vi "Fitts_test.vi"(11 "ID":dbl) -> (1 "W":dbl, 2 "D":dbl=1.0)   [LabVIEW 2010]
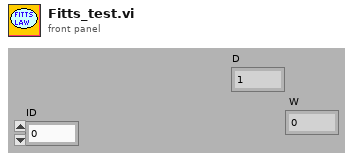
[diagram p1: front panel]
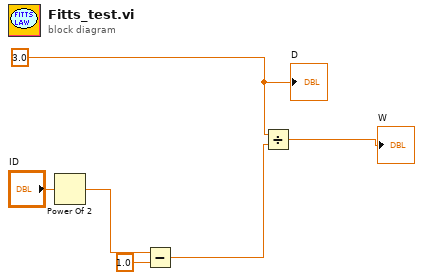
[diagram p0: block diagram]
diagram:
  w3 = 3.0 ("y")
  n1 = Power Of 2(x="ID") -> (2^x=w6:dbl)
  n2 = Subtract(x=w6, y=1.0) -> (x-y=w2:dbl)
  n3 = Divide(x=w3, y=w2) -> (x/y=→"W":dbl)
  "D" <- w3
